vi "Eth Status Write Write Enable_com.vi"(7 "Status Reference":T1, 8 "error in (no error)":errorcluster, 9 "Write Enable":bool) -> (0 "error out":errorcluster)   [LabVIEW 2021, in "Eth Status.lvlib"]
uses:
  Eth Status.lvlib
  Ctl/Status.ctl
  MB_TCP2/MB_TCP_State.ctl
  MB_TCP2/MB_TCP.lvclass
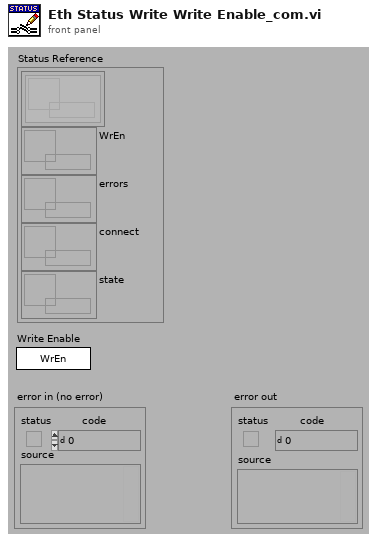
[diagram p1: front panel]
types:
  T1 = typedef "Eth Status.lvlib/Status.ctl" = cluster{"Set_states":refnum<queue>[], "WrEn":refnum<data-value>, "errors":refnum<data-value>, "connect":refnum<data-value>, "state":refnum<data-value>}
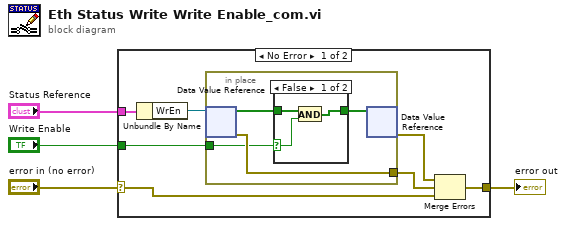
[diagram p0: block diagram]
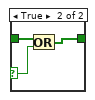
[diagram p2: hidden frame]
diagram:
  n1 = case shown="No Error" "error in (no error)" {
    selector: "error in (no error)" -> [w9 w22]
    tunnel: [w10 w22] -> w4
    tunnel: "Status Reference" -> [w11 _]
    tunnel: "Write Enable" -> [w7 _]
    frame No Error {
      n2 = Unbundle By Name(w11) -> ("WrEn"=w8:refnum<data-value>)
      n3 = in-place {
        in-place-border: [w15] -> w5
        in-place-border: w7 -> [w14]
        n4 = in-place-dvr #1(w8) -> (w13:bool[], w15:errorcluster)
        n5 = case shown="False" w14 {
          selector: w14 -> [w17 w20]
          tunnel: w13 -> [w18 w21]
          tunnel: [w16 w19] -> w12
          frame False {
            n6 = And(x=w18, y=w17) -> (x .and. y?=w16:bool[])
          }
          frame True {
            n7 = Or(x=w21, y=w20) -> (x .or. y?=w19:bool[])
          }
        }
        n8 = in-place-dvr #1(w12) -> (w6:errorcluster)  [unwired: 1 out]
      }
      n9 = Merge Errors(w6, w5, w9) -> (w10:errorcluster)
    }
    frame Error {
    }
  }
  "error out" <- w4
